vi "XML-Read-to-Array-and-Preprocessing.vi"() -> ()   [LabVIEW 2020]
panel:
  out "Output Bias (4x1)":dbl[][](array[numeric])
  out "Output Weights (4x8)":dbl[][](array[numeric])
  out "LSTM2 hidden Bias (8x4)":dbl[][](array[numeric])
  out "LSTM2 Input Bias (8x4)":dbl[][](array[numeric])
  out "LSTM2 hidden weights (32x8)":dbl[][](array[numeric])
  out "LSTM2 Input Weights (32x15)":dbl[][](array[numeric])
  out "LSTM1 hidden Bias (15x4)":dbl[][](array[numeric])
  out "LSTM1 Input Bias (15x4)":dbl[][](array[numeric])
  out "LSTM1 hidden weights (15x60)":dbl[][](array[numeric])
  out "LSTM1 Input Weights (250x60)":dbl[][](array[numeric])
  out "Input Bias (250x1)":dbl[][](array[numeric])
  out "Input Weights (250x2000)":dbl[][](array[numeric])
  out "Array":i32[](array[numeric])
  in  "test_set?":bool=TRUE
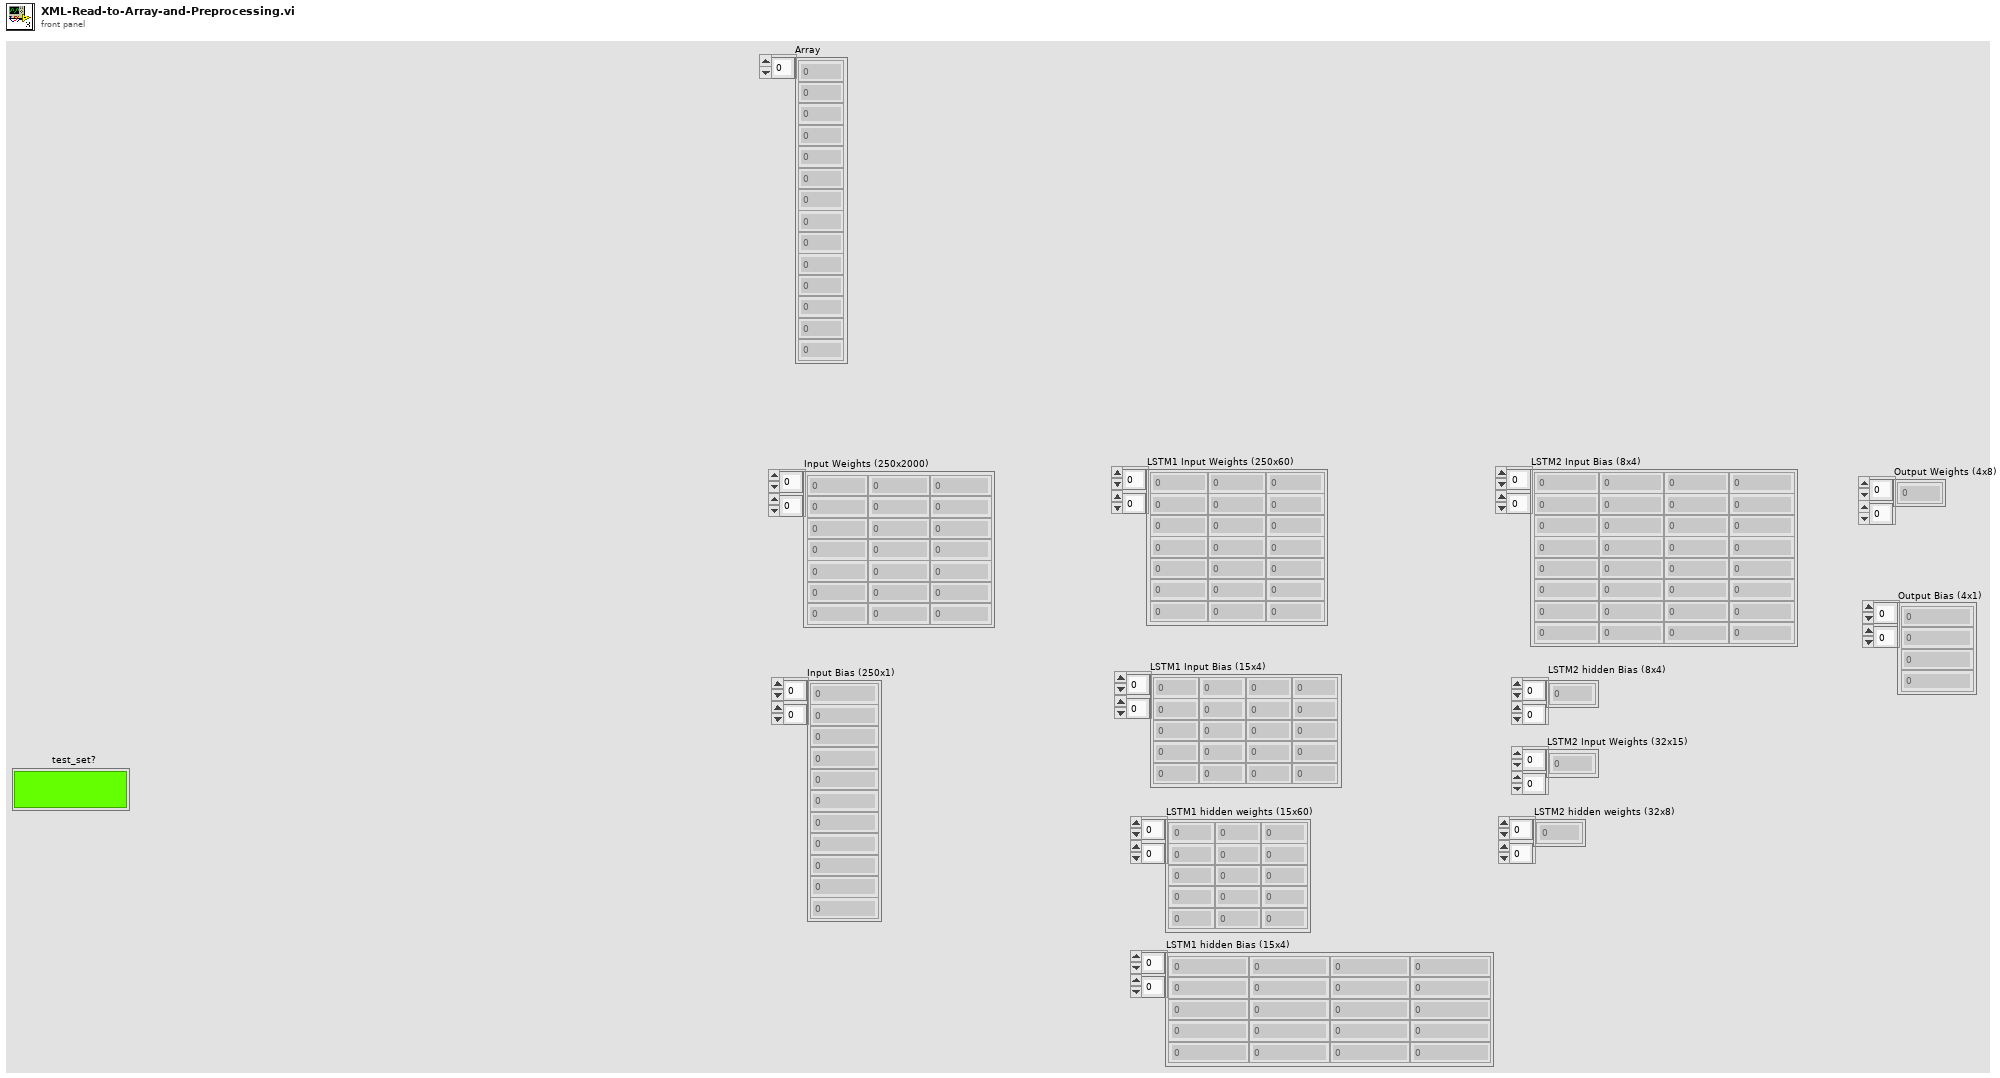
[diagram p1: front panel]
types:
  T1 = cluster{"array type (2D Dbl)":dbl[][], "array type (2D Dbl)":dbl[][], "array type (2D Dbl)":dbl[][], "array type (2D Dbl)":dbl[][], "array type (2D Dbl)":dbl[][], "array type (2D Dbl)":dbl[][], "array type (2D Dbl)":dbl[][], "array type (2D Dbl)":dbl[][], "array type (2D Dbl)":dbl[][], "array type (2D Dbl)":dbl[][], "array type (2D Dbl)":dbl[][], "array type (2D Dbl)":dbl[][]}
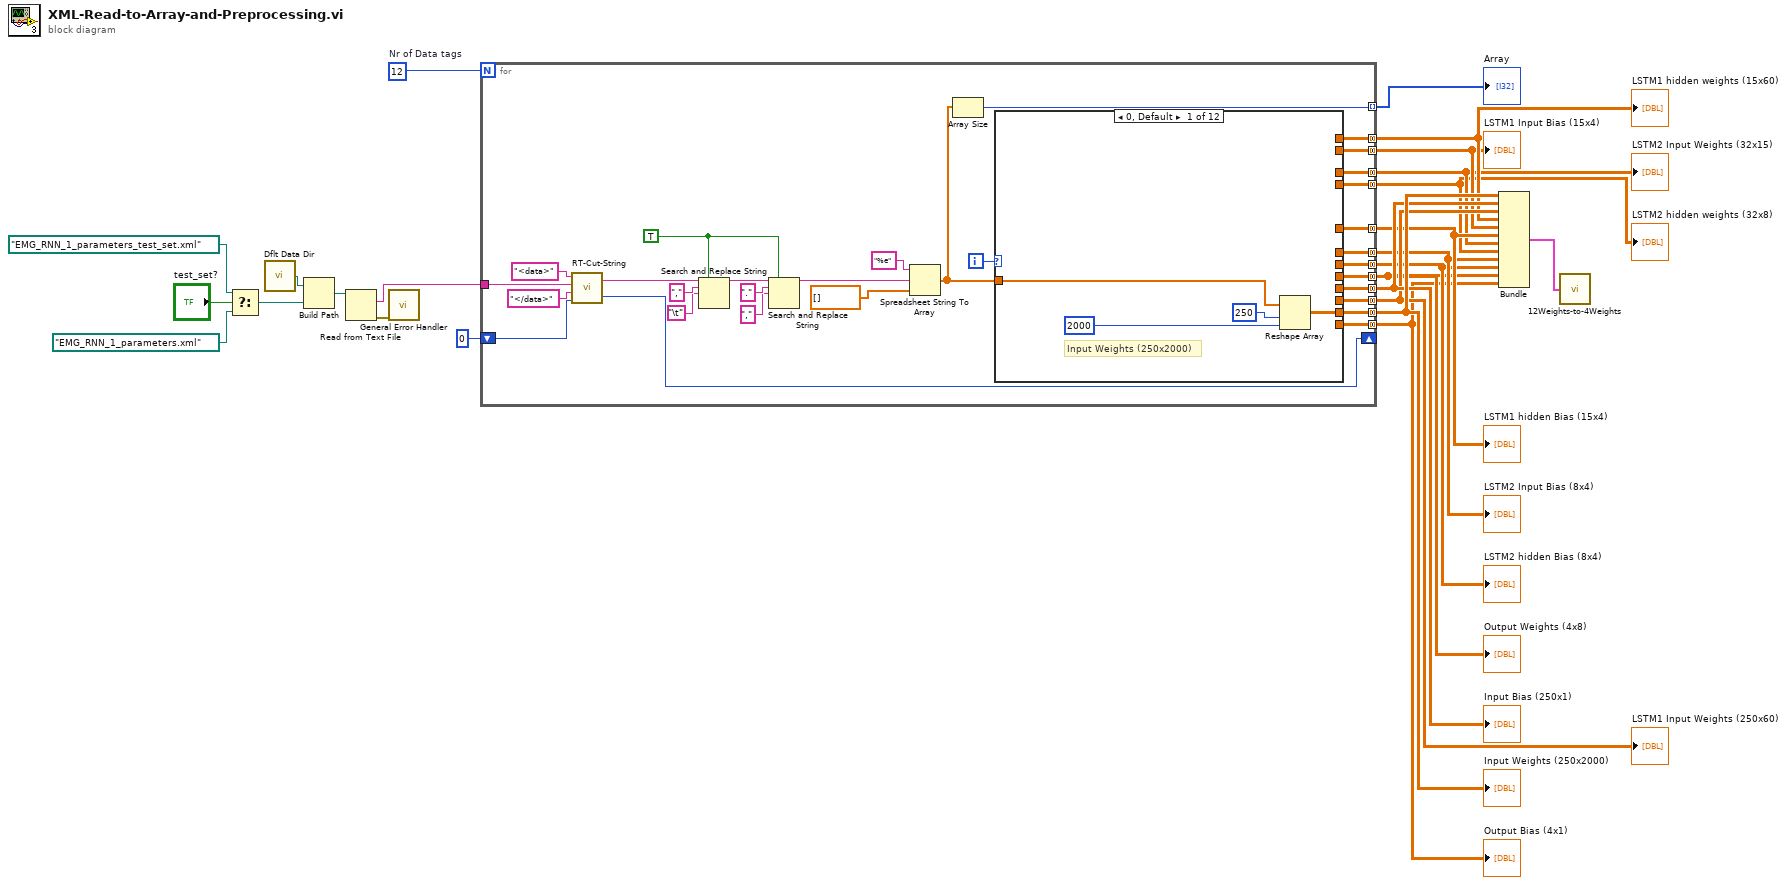
[diagram p0: block diagram]
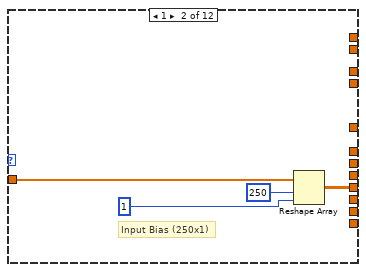
[diagram p2: hidden frame]
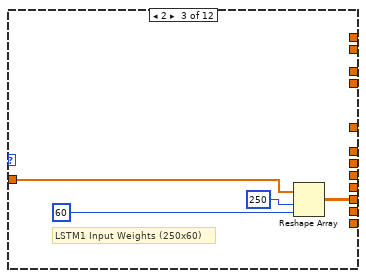
[diagram p3: hidden frame]
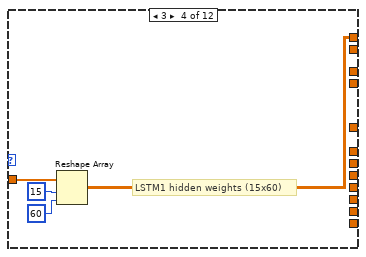
[diagram p4: hidden frame]
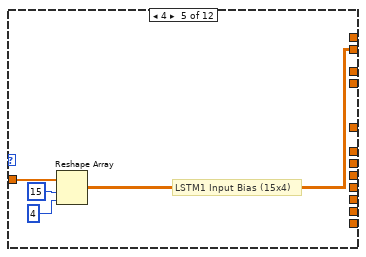
[diagram p5: hidden frame]
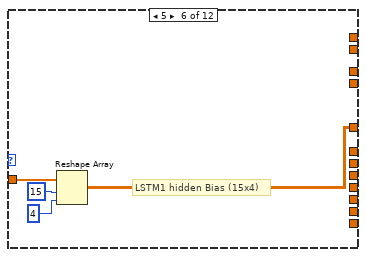
[diagram p6: hidden frame]
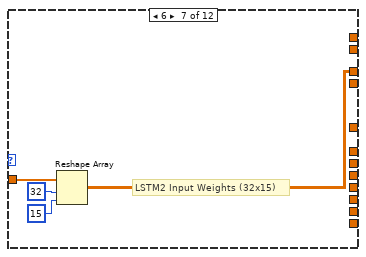
[diagram p7: hidden frame]
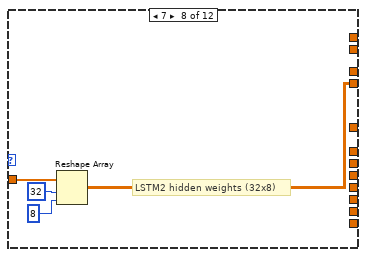
[diagram p8: hidden frame]
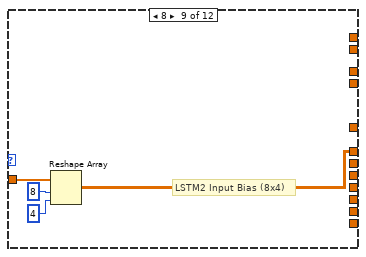
[diagram p9: hidden frame]
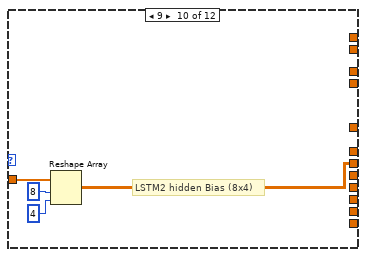
[diagram p10: hidden frame]
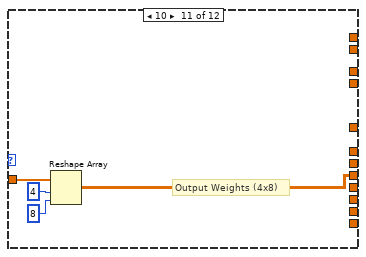
[diagram p11: hidden frame]
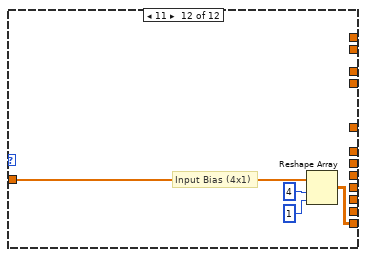
[diagram p12: hidden frame]
diagram:
  w16 = 12  # Nr of Data tags
  n1 = Select(t=path "EMG_RNN_1_parameters_test_set.xml" ("name or relative path"), s="test_set?", f=path "EMG_RNN_1_parameters.xml" ("name or relative path")) -> (s? t:f=w19:path)
  n2 = call <vilib>:"Dflt Data Dir.vi"() -> ("App:Default Data Directory"=w24:path)
  n3 = Build Path(base path=w24, name or relative path=w19) -> (appended path=w23:path)
  n4 = Read from Text File(file (use dialog)=w23) -> (text=w22:string, error out=w21:errorcluster)  [unwired: 3 in, 2 out]
  n5 = call <vilib>:"General Error Handler.vi"("error in (no error)"=w21) -> ()  [unwired: 10 in, 5 out]
  n6 = for {
    N: w16 -> [_]
    tunnel: w22 -> [w53]
    shift-right: [w50] -> _
    shift-left: 0 ("offset past match") -> [w51]
    tunnel: [w37] -> w14 mode=indexing
    tunnel: [w36] -> w13 mode=concatenating
    tunnel: [w35] -> w12 mode=concatenating
    tunnel: [w34] -> w11 mode=concatenating
    tunnel: [w33] -> w10 mode=concatenating
    tunnel: [w32] -> w9 mode=concatenating
    tunnel: [w31] -> w8 mode=concatenating
    tunnel: [w30] -> w7 mode=concatenating
    tunnel: [w29] -> w6 mode=concatenating
    tunnel: [w28] -> w5 mode=concatenating
    tunnel: [w27] -> w4 mode=concatenating
    tunnel: [w26] -> w3 mode=concatenating
    tunnel: [w25] -> w2 mode=concatenating
    i -> [w39]
    w40 = TRUE ("replace all? (F)")
    n7 = call "RT-Cut-String.vi"("offset (0)"=w51, "End Cut"="</data>", "Input string"=w53, "Start Cut"="<data>") -> ("offset past match"=w50:i32, "Extracted"=w42:string)
    n8 = Search and Replace String(replace all?=w40, input string=w42, search string="," ("search string/char (-)"), replace string="\t") -> (result string=w47:string)  [unwired: 4 in, 3 out]
    n9 = Search and Replace String(replace all?=w40, input string=w47, search string="." ("search string/char (-)"), replace string="," ("search string/char (-)")) -> (result string=w41:string)  [unwired: 4 in, 3 out]
    n10 = Spreadsheet String To Array(format string="%e", spreadsheet string=w41, array type (2D Dbl)=dbl[] []) -> (array=w38:dbl[])  [unwired: 1 in]
    n11 = Array Size(array=w38) -> (size(s)=w37:i32)
    n12 = case shown="0, Default" w39 {
      tunnel: w38 -> [w55 w60 w64 w67 w71 w75 w79 w83 w87 w91 w95 w100]
      tunnel: [w56 _ _ _ _ _ _ _ _ _ _ _] -> w36
      tunnel: [_ w59 _ _ _ _ _ _ _ _ _ _] -> w35
      tunnel: [_ _ w63 _ _ _ _ _ _ _ _ _] -> w34
      tunnel: [_ _ _ w68 _ _ _ _ _ _ _ _] -> w33
      tunnel: [_ _ _ _ w72 _ _ _ _ _ _ _] -> w32
      tunnel: [_ _ _ _ _ w76 _ _ _ _ _ _] -> w31
      tunnel: [_ _ _ _ _ _ w80 _ _ _ _ _] -> w30
      tunnel: [_ _ _ _ _ _ _ w84 _ _ _ _] -> w29
      tunnel: [_ _ _ _ _ _ _ _ w88 _ _ _] -> w28
      tunnel: [_ _ _ _ _ _ _ _ _ w92 _ _] -> w27
      tunnel: [_ _ _ _ _ _ _ _ _ _ w96 _] -> w26
      tunnel: [_ _ _ _ _ _ _ _ _ _ _ w99] -> w25
      frame 0, Default {
        # "Input Weights (250x2000)"
        n13 = Reshape Array(w55, 250 ("dimension size"), 2000 ("dimension size")) -> (w56:dbl[][])
      }
      frame 1 {
        # "Input Bias (250x1)"
        n14 = Reshape Array(w60, 250 ("dimension size"), 1 ("dimension size")) -> (w59:dbl[][])
      }
      frame 2 {
        # "LSTM1 Input Weights (250x60)"
        n15 = Reshape Array(w64, 250 ("dimension size"), 60 ("dimension size")) -> (w63:dbl[][])
      }
      frame 3 {
        # "LSTM1 hidden weights (15x60)"
        n16 = Reshape Array(w67, 15 ("dimension size"), 60 ("dimension size")) -> (w68:dbl[][])
      }
      frame 4 {
        # "LSTM1 Input Bias (15x4)"
        n17 = Reshape Array(w71, 15 ("dimension size"), 4 ("dimension size")) -> (w72:dbl[][])
      }
      frame 5 {
        # "LSTM1 hidden Bias (15x4)"
        n18 = Reshape Array(w75, 15 ("dimension size"), 4 ("dimension size")) -> (w76:dbl[][])
      }
      frame 6 {
        # "LSTM2 Input Weights (32x15)"
        n19 = Reshape Array(w79, 32 ("dimension size"), 15 ("dimension size")) -> (w80:dbl[][])
      }
      frame 7 {
        # "LSTM2 hidden weights (32x8)"
        n20 = Reshape Array(w83, 32 ("dimension size"), 8 ("dimension size")) -> (w84:dbl[][])
      }
      frame 8 {
        # "LSTM2 Input Bias (8x4)"
        n21 = Reshape Array(w87, 8 ("dimension size"), 4 ("dimension size")) -> (w88:dbl[][])
      }
      frame 9 {
        # "LSTM2 hidden Bias (8x4)"
        n22 = Reshape Array(w91, 8 ("dimension size"), 4 ("dimension size")) -> (w92:dbl[][])
      }
      frame 10 {
        # "Output Weights (4x8)"
        n23 = Reshape Array(w95, 4 ("dimension size"), 8 ("dimension size")) -> (w96:dbl[][])
      }
      frame 11 {
        # "Input Bias (4x1)"
        n24 = Reshape Array(w100, 4 ("dimension size"), 1 ("dimension size")) -> (w99:dbl[][])
      }
    }
  }
  "Array" <- w14
  "Input Weights (250x2000)" <- w13
  "Input Bias (250x1)" <- w12
  "LSTM1 Input Weights (250x60)" <- w11
  "LSTM1 hidden weights (15x60)" <- w10
  "LSTM1 Input Bias (15x4)" <- w9
  "LSTM1 hidden Bias (15x4)" <- w8
  "LSTM2 Input Weights (32x15)" <- w7
  "LSTM2 hidden weights (32x8)" <- w6
  "LSTM2 Input Bias (8x4)" <- w5
  "LSTM2 hidden Bias (8x4)" <- w4
  "Output Weights (4x8)" <- w3
  "Output Bias (4x1)" <- w2
  n25 = Bundle("array type (2D Dbl)"=w13, "array type (2D Dbl)"=w12, "array type (2D Dbl)"=w11, "array type (2D Dbl)"=w10, "array type (2D Dbl)"=w9, "array type (2D Dbl)"=w8, "array type (2D Dbl)"=w7, "array type (2D Dbl)"=w6, "array type (2D Dbl)"=w5, "array type (2D Dbl)"=w4, "array type (2D Dbl)"=w3, "array type (2D Dbl)"=w2) -> (w1:T1)  [unwired: 1 in]
  n26 = call "12Weights-to-4Weights.vi"("output cluster"=w1) -> ()
